vi "primary control loop.vi"(8 "loop comms in":T1, 9 "worker pool reference":T17, 10 "cmd fifo":refnum<k33>, 11 "engine out":T2={"timed loop timer source"={"Processor"=-2, "Priority"=0, "timing source dt"=0, "timer source"=refnum}, "control loop data"={"engine tag bus"={"Double"=[], "Single"=[], "I64"=[], "I32"=[], "I16"=[], "I8"=[], "U64"=[], "U32"=[], "U16"=[], "U8"=[], "Boolean"=[], "String"=[], "Array of Double"=[], "Array of Single"=[], "Array of I64"=[], "Array of I32"=[], "Array of I16"=[], "Array of I8"=[], "Array of U64"=[], "Array of U32"=[], "Array of U16"=[], "Array of U8"=[], "Array of Boolean"=[], "Array of String"=[]}, "engine schedule"={"module run flags"=[], "decimation schedule"={"decimations"=[], "offsets"=[]}}, "module information"=[]}, "status reporting"={"late? index (bool)"=-1, "late count index (U32)"=-1, "dt (ns) index (U64)"=-1, "execution time (ns) index (U64)"=-1}}) -> (0 "error out":errorcluster, 2 "desired state":T20, 3 "engine out":T2={"timed loop timer source"={"Processor"=-2, "Priority"=0, "timing source dt"=0, "timer source"=refnum}, "control loop data"={"engine tag bus"={"Double"=[], "Single"=[], "I64"=[], "I32"=[], "I16"=[], "I8"=[], "U64"=[], "U32"=[], "U16"=[], "U8"=[], "Boolean"=[], "String"=[], "Array of Double"=[], "Array of Single"=[], "Array of I64"=[], "Array of I32"=[], "Array of I16"=[], "Array of I8"=[], "Array of U64"=[], "Array of U32"=[], "Array of U16"=[], "Array of U8"=[], "Array of Boolean"=[], "Array of String"=[]}, "engine schedule"={"module run flags"=[], "decimation schedule"={"decimations"=[], "offsets"=[]}}, "module information"=[]}, "status reporting"={"late? index (bool)"=-1, "late count index (U32)"=-1, "dt (ns) index (U64)"=-1, "execution time (ns) index (U64)"=-1}})   [LabVIEW 2013, in "main engine.lvlib"]
doc: "Runs the main control timed loop of the engine."
uses:
  main engine.lvlib
  <vilib>/NI/DCAF Execution Engine Interface/Engine Runtime/Execution States.ctl
  worker library/worker comms.ctl
  worker library/worker commands.ctl
  worker library/request fifos.ctl
  worker library/recovery request.ctl
  <vilib>/NI/DCAF Module Framework/runtime/TBM module execution interface.lvclass
  <vilib>/NI/DCAF Module Framework/module configuration/TBM module configuration.lvclass
  worker library/rt fault.ctl
  <vilib>/NI/DCAF Module Framework/runtime/error classification.ctl
  worker library/response fifos.ctl
  worker library/recovery response.ctl
  <vilib>/NI/DCAF Execution Engine Interface/Engine Runtime/Fault.ctl
  Engine Data.ctl
  <vilib>/NI/Module Timing Source/timing source/TBM timing source.lvclass
  timed loop timing sources.ctl
  control loop data.ctl
  <vilib>/NI/Tag Bus/table/data table.ctl
  engine run schedule.ctl
  engine decimation schedule.ctl
  full module data.ctl
  module run state.ctl
  async executor/asynchronous executor reference.ctl
  async executor/async message to executor.ctl
  Runtime/async command notification.ctl
  Runtime/async error info.ctl
  module method data.ctl
  <vilib>/NI/Tag Bus/table/transfer specification.ctl
  <vilib>/NI/Tag Bus/tag/Data Type.ctl
  fault handling spec.ctl
  Configuration/Error Actions.ctl
  status reporting data.ctl
  loop comms.ctl
  message to engine.ctl
  message request type.ctl
  message from engine.ctl
  message response type.ctl
  <vilib>/Platform/TimedLoop/XDataNode/timing_clust.ctl
  <vilib>/Platform/TimedLoop/XDataNode/nitl_modes.ctl
  <vilib>/Platform/TimedLoop/XDataNode/wakeup.ctl
  time information.ctl
  <vilib>/NI/Tag Bus/table/transfer table data.vi
  async executor/async input data method.vi
  async executor/async process data method.vi
  async executor/async output data method.vi
  <vilib>/platform/TimedLoop/XDataNode/XDataNode.xnode
  <vilib>/Platform/TimedLoop/XDataNode/XDNodeRunTimeDep.lvlib
  <vilib>/NI/DCAF Execution Engine Interface/Engine Runtime/Engine Runtime Interface.lvclass
  <vilib>/NI/Tag Bus/table/data table.lvlib
  <vilib>/NI/Tag Bus/tag/tag descriptor.lvclass
  Configuration/Standard Engine Configuration.lvclass
  worker library/worker pool.lvlib
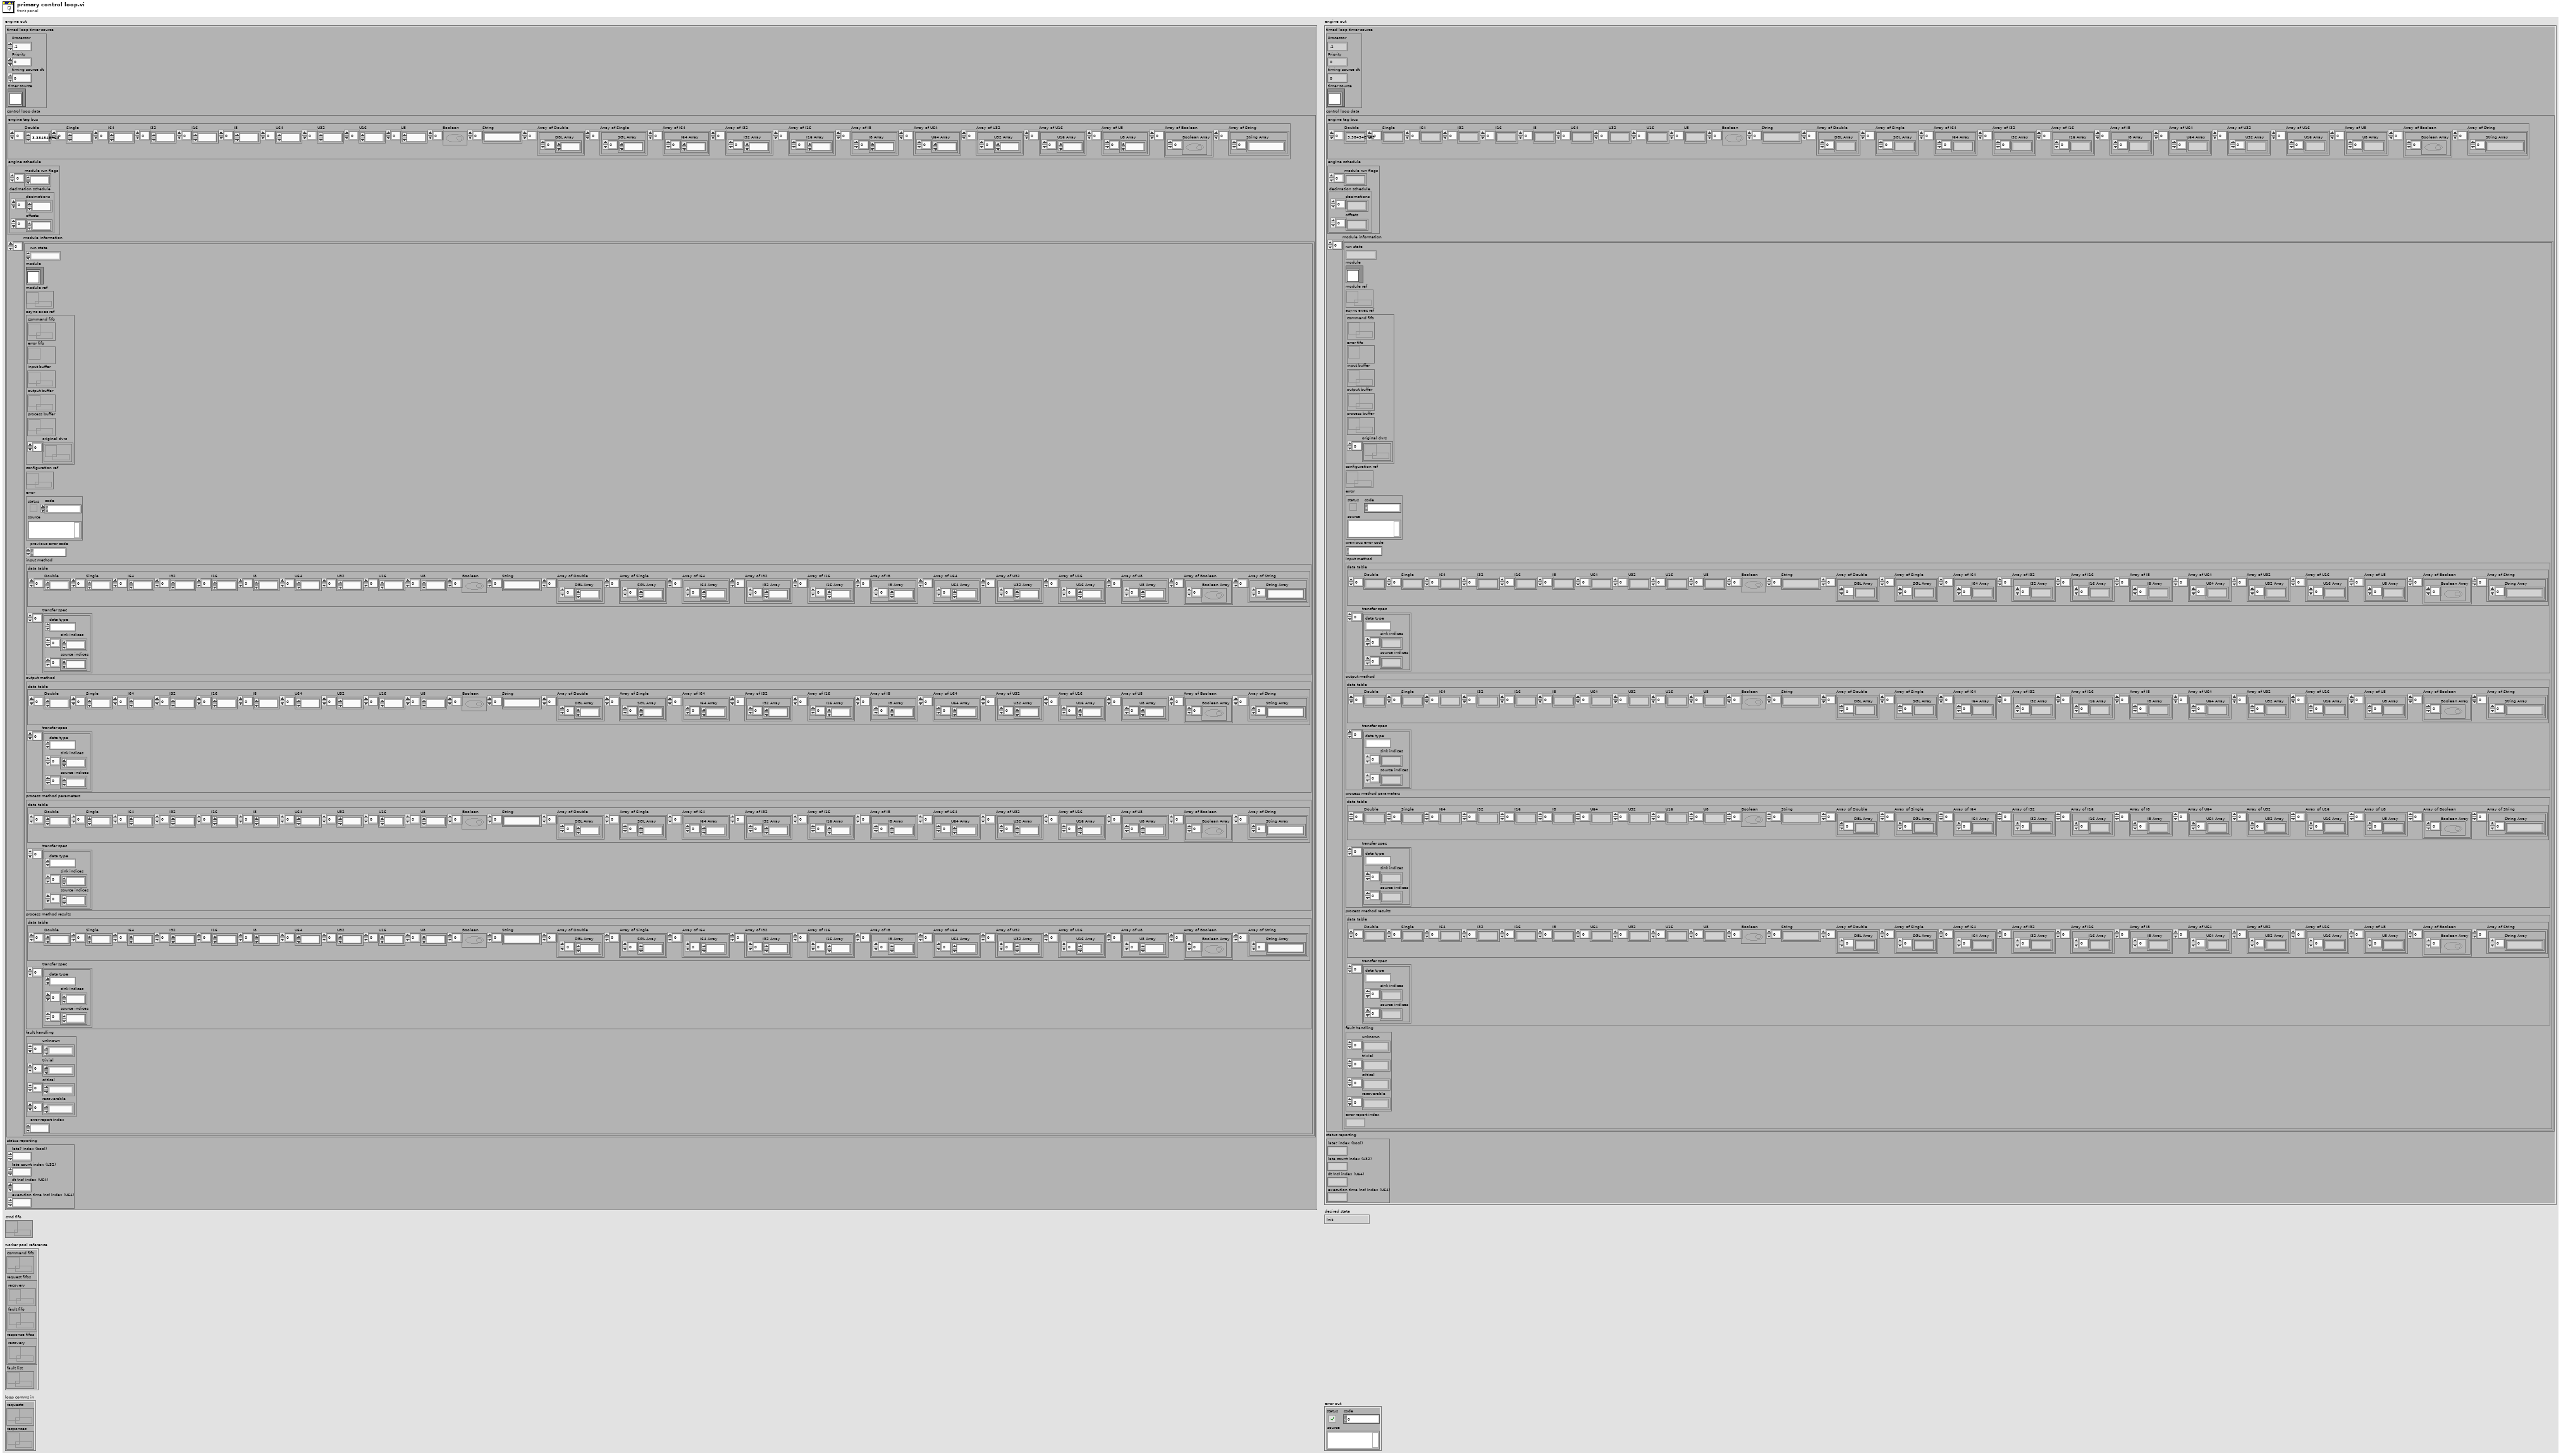
[diagram p1: front panel]
types:
  T1 = typedef "main engine.lvlib/loop comms.ctl" = cluster{"requests":refnum<k33>, "responses":refnum<k33>}
  T2 = typedef "main engine.lvlib/Engine Data.ctl" = cluster{"timed loop timer source":T3, "control loop data":T4, "status reporting":T16}
  T3 = typedef "main engine.lvlib/timed loop timing sources.ctl" = cluster{"Processor":i32, "Priority":i32, "timing source dt":u32, "timer source":refnum<class "TBM timing source.lvclass">}
  T4 = typedef "main engine.lvlib/control loop data.ctl" = cluster{"engine tag bus":T5, "engine schedule":T6, "module information":T8[]}
  T5 = typedef "tag bus.lvlib/data table.lvlib/data table.ctl" = cluster{"Double":dbl[], "Single":sgl[], "I64":i64[], "I32":i32[], "I16":i16[], "I8":i8[], "U64":u64[], "U32":u32[], "U16":u16[], "U8":u8[], "Boolean":bool[], "String":string[], "Array of Double":cluster{"DBL Array":dbl[]}[], "Array of Single":cluster{"SGL Array":sgl[]}[], "Array of I64":cluster{"I64 Array":i64[]}[], "Array of I32":cluster{"I32 Array":i32[]}[], "Array of I16":cluster{"I16 Array":i16[]}[], "Array of I8":cluster{"I8 Array":i8[]}[], "Array of U64":cluster{"U64 Array":u64[]}[], "Array of U32":cluster{"U32 Array":u32[]}[], "Array of U16":cluster{"U16 Array":u16[]}[], "Array of U8":cluster{"U8 Array":u8[]}[], "Array of Boolean":cluster{"Boolean Array":bool[]}[], "Array of String":cluster{"String Array":string[]}[]}
  T6 = typedef "main engine.lvlib/engine run schedule.ctl" = cluster{"module run flags":u8[], "decimation schedule":T7}
  T7 = typedef "main engine.lvlib/engine decimation schedule.ctl" = cluster{"decimations":u16[], "offsets":u16[]}
  T8 = typedef "main engine.lvlib/full module data.ctl" = cluster{"run state":T9, "module":refnum<class "TBM module execution interface.lvclass">, "module ref":refnum<data-value>, "async exec ref":T10, "configuration ref":refnum<data-value>, "error":errorcluster, "previous error code":i32, "input method":T11, "output method":T11, "process method parameters":T11, "process method results":T11, "fault handling":T14, "error report index ":i32}
  T9 = typedef "main engine.lvlib/module run state.ctl" = enum16{"sync", "async"}
  T10 = typedef "main engine.lvlib/asynchronous executor reference.ctl" = cluster{"command fifo":refnum<k33>, "error fifo":refnum<k33>, "input buffer":refnum<k33>, "output buffer":refnum<k33>, "process buffer":refnum<k33>, "original dvrs":refnum<data-value>[]}
  T11 = typedef "main engine.lvlib/module method data.ctl" = cluster{"data table":T5, "transfer spec":T12[]}
  T12 = typedef "tag bus.lvlib/data table.lvlib/transfer specification.ctl" = cluster{"data type":T13, "sink indices":i32[], "source indices":i32[]}
  T13 = typedef "tag bus.lvlib/tag descriptor.lvclass/Data Type.ctl" = enum16{"Double", "Single", "I64", "I32", "I16", "I8", "U64", "U32", "U16", "U8", "Boolean", "String", "Array of Double", "Array of Single", "Array of I64", "Array of I32", "Array of I16", "Array of I8", "Array of U64", "Array of U32", "Array of U16", "Array of U8", "Array of Boolean", "Array of String"}
  T14 = typedef "main engine.lvlib/fault handling spec.ctl" = cluster{"unknown":T15[], "trivial":T15[], "critical":T15[], "recoverable":T15[]}
  T15 = typedef "Standard Engine Configuration.lvclass/Error Actions.ctl" = enum16{"Clear", "Notify", "Stop Component", "Stop Engine", "Safe State", "Attempt Recovery"}
  T16 = typedef "main engine.lvlib/status reporting data.ctl" = cluster{"late? index (bool)":i32, "late count index (U32)":i32, "dt (ns) index (U64)":i32, "execution time (ns) index (U64)":i32}
  T17 = typedef "worker pool.lvlib/worker comms.ctl" = cluster{"command fifo":refnum<k33>, "request fifos":T18, "response fifos":T19, "fault list":refnum<data-value>}
  T18 = typedef "worker pool.lvlib/request fifos.ctl" = cluster{"recovery":refnum<k33>, "fault fifo":refnum<k33>}
  T19 = typedef "worker pool.lvlib/response fifos.ctl" = cluster{"recovery":refnum<k33>}
  T20 = typedef "Engine Runtime Interface.lvclass/Execution States.ctl" = enum16{"Init", "Pre-Operational", "Safe-Operational", "Operational", "Stopped"}
  T21 = typedef "main engine.lvlib/time information.ctl" = cluster{"ns since last call":u64, "finished late?":bool, "late count":u32, "iterations":u64, "ns exec time":u64}
  T22 = typedef "XDNodeRunTimeDep.lvlib/timing_clust.ctl" = cluster{"Expected End [f-1]":u64, "Actual End [f-1]":u64, "Finished Late? [f-1]":bool, "Expected End [i-1]":u64, "Actual End [i-1]":u64, "Finished Late? [i-1]":bool, "Expected Start [i]":u64, "Actual Start [i]":u64, "Expected Start [f]":u64, "Actual Start [f]":u64, "Source Name":string, "Structure Name":string, "Period":i64, "Deadline":i64, "Offset":i64, "Start":i64, "Priority":i32, "Timeout":i32, "Mode":T23, "Wakeup Reason":T24, "Error":errorcluster, "Source Type":string, "Secondary Source Type":string, "Global End Time":u64, "Global Start Time":u64, "Frame Duration":u64, "Iteration Duration":u64, "Assigned CPU":i32, "I/O Scan Engine Mode":u32}
  T23 = typedef "XDNodeRunTimeDep.lvlib/nitl_modes.ctl" = enum32{"No Change", "Process missed periods, maintain original phase", "Discard missed periods, maintain original phase", "Process missed periods, ignore original phase", "Discard missed periods, ignore original phase"}
  T24 = typedef "XDNodeRunTimeDep.lvlib/wakeup.ctl" = enum32{"Normal", "Aborted", "Asynchronous wakeup", "Timing source error", "Timed loop error", "Timeout"}
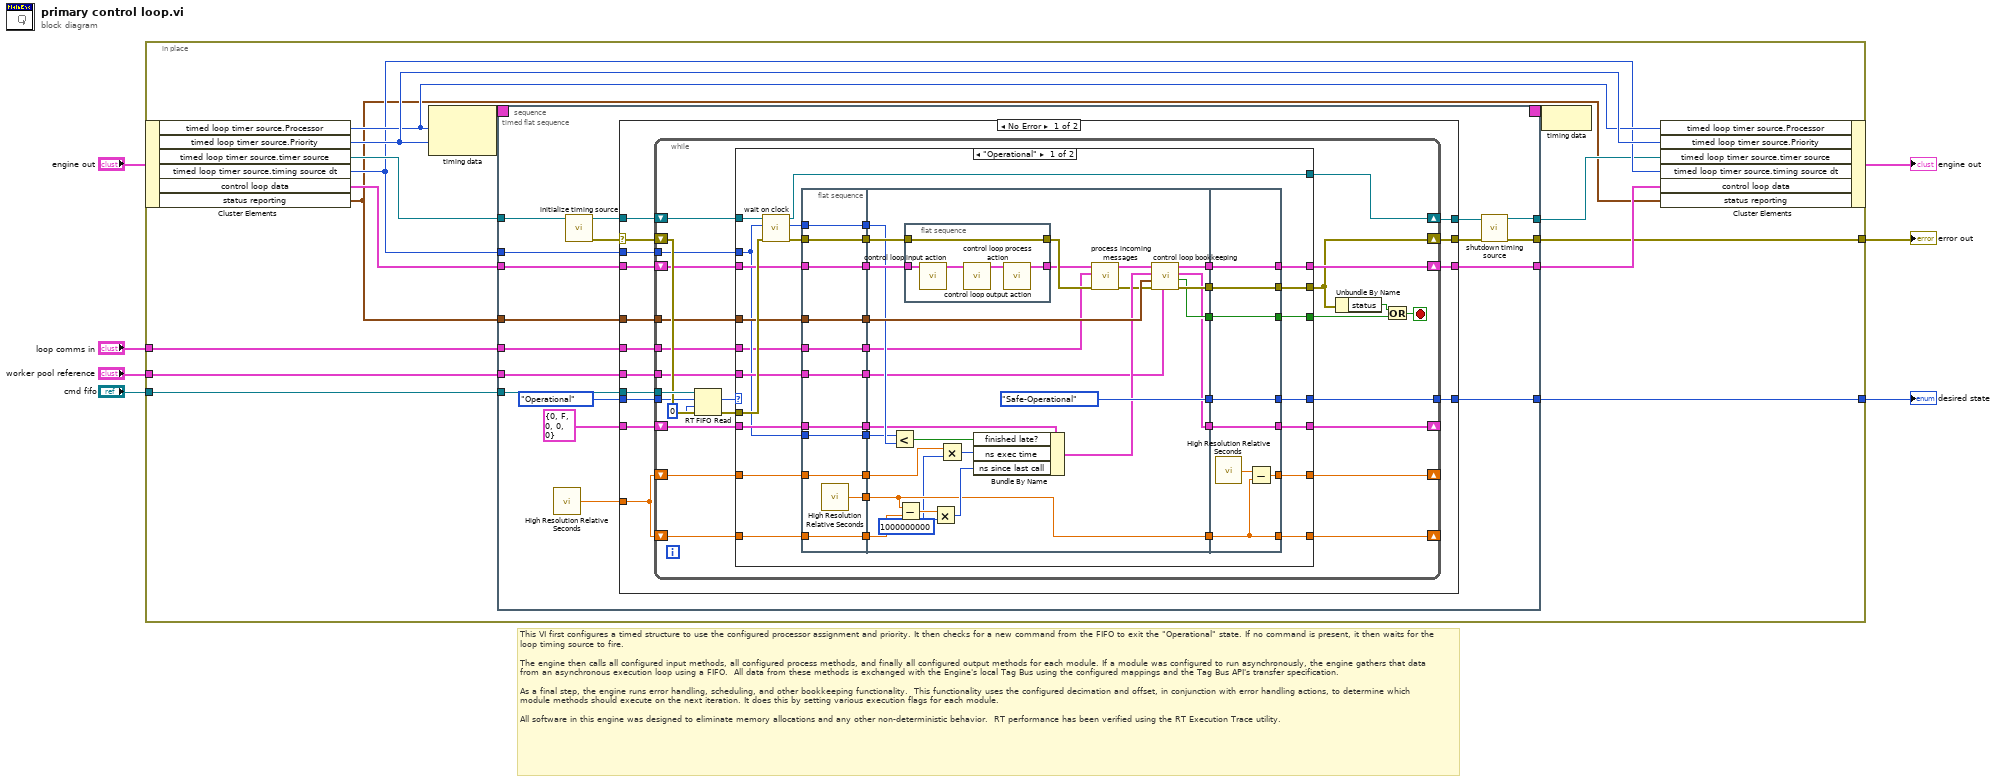
[diagram p0: block diagram]
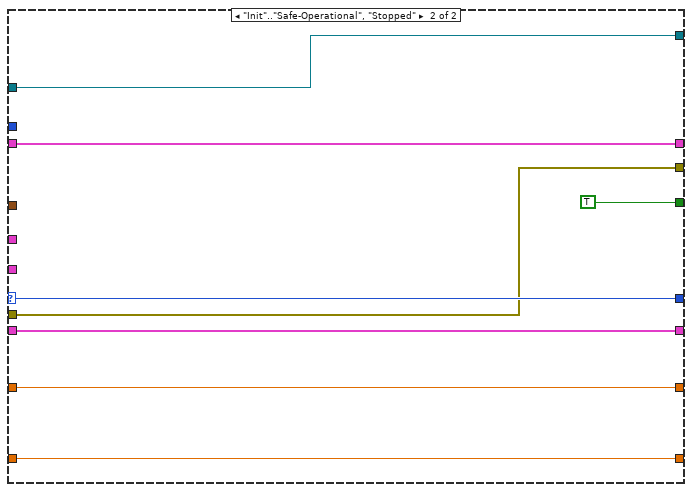
[diagram p2: hidden frame]
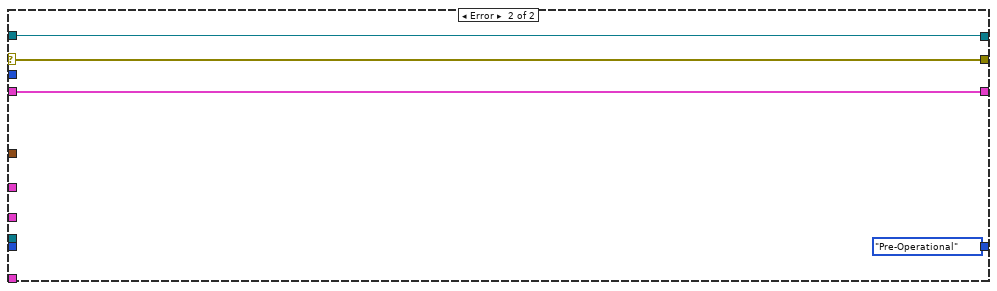
[diagram p3: hidden frame]
diagram:
  # "This VI first configures a timed structure to use the configured processor assignment and priority. It then checks for a new command from the FIFO to exit the \"Operational\" state. If no command is present, it then waits for the loop timing source to fire.   \n\nThe engine then calls all configured input methods, all configured process methods, and finally all configured output methods for each module. If a module was configured to run asynchronously, the engine gathers that data from an asynchronous execution loop using a FIFO.  All data from these methods is exchanged with the Engine's local Tag Bus using the configured mappings and the Tag Bus API's transfer specification. \n\nAs a final step, the engine runs error handling, scheduling, and other bookkeeping functionality.  This functionality uses the configured decimation and offset, in conjunction with error handling actions, to determine which module methods should execute on the next iteration. It does this by setting various execution flags for each module.\n\nAll software in this engine was designed to eliminate memory allocations and any other non-deterministic behavior.  RT performance has been verified using the RT Execution Trace utility."
  n1 = in-place {
    in-place-border: [w13] -> w5
    in-place-border: "cmd fifo" -> [w12]
    in-place-border: "worker pool reference" -> [w11]
    in-place-border: [w10] -> w2
    in-place-border: "loop comms in" -> [w8]
    n2 = in-place-cluster #1("engine out") -> ("timed loop timer source.Processor"=w17:i32, "timed loop timer source.Priority"=w18:i32, "timed loop timer source.timer source"=w20:refnum<class "TBM timing source.lvclass">, "timed loop timer source.timing source dt"=w16:u32, "control loop data"=w19:T4, "status reporting"=w9:T16)
    n3 = node-c288(w17, w18) -> (w22:T22)
    n4 = timed-sequence {
      timing: w22 -> [_]
      timing-out: [_] -> w21
      tunnel: w20 -> [w33]
      tunnel: w19 -> [w28]
      tunnel: w16 -> [w32]
      tunnel: [w31] -> w15
      tunnel: [w30] -> w13
      tunnel: [w29] -> w14
      tunnel: w12 -> [w27]
      tunnel: w11 -> [w26]
      tunnel: [w25] -> w10
      tunnel: w9 -> [w24]
      tunnel: w8 -> [w23]
      n5 = timed-flat-sequence {
        tunnel: w33 -> [w51]
        tunnel: w32 -> [w49]
        tunnel: [w42] -> w31
        tunnel: [w44] -> w30
        tunnel: [w46] -> w29
        tunnel: w28 -> [w45]
        tunnel: w27 -> [w41]
        tunnel: w26 -> [w40]
        tunnel: [w38] -> w25
        tunnel: w24 -> [w37]
        tunnel: w23 -> [w34]
        n6 = call <vilib>:"High Resolution Relative Seconds.vi"() -> ("relative seconds"=w36:dbl)
        n7 = call-dynamic "initialize timing source.vi"("timing source in"=w51) -> ("error out"=w50:errorcluster, "timing source out"=w48:refnum<class "TBM timing source.lvclass">)  [unwired: 9 in]
        n8 = case shown="No Error" w50 {
          selector: w50 -> [w64 w189]
          tunnel: w49 -> [w56 _]
          tunnel: [w65 w190] -> w43
          tunnel: w48 -> [w66 w190]
          tunnel: [w63 w189] -> w47
          tunnel: [w61 w188] -> w46
          tunnel: w45 -> [w62 w188]
          tunnel: w41 -> [w60 _]
          tunnel: w40 -> [w59 _]
          tunnel: Execution_States."Operational" ("element") -> [w58 _]
          tunnel: [w57 Execution_States."Pre-Operational"] -> w38
          tunnel: w37 -> [w55 _]
          tunnel: w36 -> [w53 _]
          tunnel: T21 {"ns since last call"=0, "finished late?"=FALSE, "late count"=0, "iterations"=0, "ns exec time"=0} ("time data") -> [w54 _]
          tunnel: w34 -> [w52 _]
          frame No Error {
            n9 = while {
              shift-right: [w82] -> w65
              shift-left: w66 -> [w83]
              shift-right: [w76] -> w63
              shift-left: w64 -> [w90]
              shift-right: [w80] -> w61
              shift-left: w62 -> [w81]
              tunnel: w60 -> [w91]
              tunnel: w59 -> [w78]
              tunnel: w58 -> [w88]
              tunnel: [w85] -> w57
              tunnel: w56 -> [w79]
              tunnel: w55 -> [w74]
              shift-right: [w72] -> _
              shift-left: w54 -> [w73]
              shift-right: [w70] -> _
              shift-left: w53 -> [w71]
              shift-right: [w69] -> _
              shift-left: w53 -> [w68]
              tunnel: w52 -> [w67]
              stop <- w77 stop-if-true
              n10 = RT FIFO Read(0:w91, 1:w88, 2:0 ("timeout in ms (0)"), 3:w90) -> (9:w87:T20, 11:w86:errorcluster)  [unwired: 3 out]
              n11 = case shown="\"Operational\"" w87 {
                selector: w87 -> [_ w186]
                tunnel: w86 -> [w127 w185]
                tunnel: [w118 w186] -> w85
                tunnel: [w120 w185] -> w76
                tunnel: [w119 TRUE] -> w84
                tunnel: w83 -> [w128 w183]
                tunnel: [w126 w183] -> w82
                tunnel: w81 -> [w125 w182]
                tunnel: [w124 w182] -> w80
                tunnel: w79 -> [w113 _]
                tunnel: w78 -> [w114 _]
                tunnel: w74 -> [w122 _]
                tunnel: w73 -> [w117 w181]
                tunnel: [w116 w181] -> w72
                tunnel: w71 -> [w115 w180]
                tunnel: [w103 w180] -> w70
                tunnel: [w96 w179] -> w69
                tunnel: w68 -> [w95 w179]
                tunnel: w67 -> [w92 _]
                frame "Operational" {
                  n12 = call-dynamic "wait on clock.vi"("error in"=w127, "dt"=w113, "timing source in"=w128) -> ("error out"=w123:errorcluster, "ticks since last call"=w121:u32, "timing source out"=w126:refnum<class "TBM timing source.lvclass">)  [unwired: 6 in]
                  n13 = flat-sequence {
                    tunnel: w114 -> [w132]
                    tunnel: w115 -> [w133]
                    tunnel: w117 -> [w134]
                    tunnel: w113 -> [w135]
                    tunnel: w121 -> [w136]
                    tunnel: w122 -> [w137]
                    tunnel: w123 -> [w138]
                    tunnel: w125 -> [w139]
                    tunnel: [w139] -> w112
                    tunnel: [w138] -> w111
                    tunnel: [w137] -> w110
                    tunnel: [w136] -> w109
                    tunnel: [w135] -> w108
                    tunnel: [w134] -> w107
                    tunnel: [w133] -> w106
                    tunnel: [w131] -> w105
                    tunnel: [w132] -> w104
                    tunnel: w95 -> [w130]
                    tunnel: [w130] -> w94
                    tunnel: [w129] -> w93
                    tunnel: w92 -> [w129]
                    tunnel: w112 -> [w165]
                    tunnel: w111 -> [w163]
                    tunnel: w110 -> [w162]
                    tunnel: w109 -> [w161]
                    tunnel: w108 -> [w160]
                    tunnel: w107 -> [w156]
                    tunnel: w106 -> [w152]
                    tunnel: w105 -> [w148]
                    tunnel: w104 -> [w149]
                    tunnel: [w164] -> w102
                    tunnel: [w159] -> w101
                    tunnel: [w158] -> w100
                    tunnel: [Execution_States."Safe-Operational"] -> w99
                    tunnel: [w155] -> w98
                    tunnel: [w148] -> w97
                    tunnel: w94 -> [w145]
                    tunnel: w93 -> [w140]
                    tunnel: [w172] -> w103
                    tunnel: [w174] -> w116
                    tunnel: [w175] -> w118
                    tunnel: [w176] -> w119
                    tunnel: [w177] -> w120
                    tunnel: [w178] -> w124
                    tunnel: w102 -> [w178]
                    tunnel: w101 -> [w177]
                    tunnel: w100 -> [w176]
                    tunnel: w99 -> [w175]
                    tunnel: w98 -> [w174]
                    tunnel: w97 -> [w172]
                    tunnel: [w171] -> w96
                    frame #0 {
                      n14 = call <vilib>:"High Resolution Relative Seconds.vi"() -> ("relative seconds"=w131:dbl)
                    }
                    frame #1 {
                      w146 = 1000000000
                      n15 = Less?(x=w160, y=w161) -> (x < y?=w153:bool)
                      n16 = Subtract(x=w148, y=w152) -> (x-y=w151:dbl)
                      n17 = flat-sequence {
                        tunnel: w165 -> [w168]
                        tunnel: [w167] -> w143
                        tunnel: w163 -> [w166]
                        tunnel: [w166] -> w144
                        frame #0 {
                          n18 = call "control loop input action.vi"("control loop data in"=w168) -> ("control loop data out"=w170:T4)  [unwired: 10 in]
                          n19 = call "control loop process action.vi"("control loop data in"=w170) -> ("control loop data out"=w169:T4)  [unwired: 10 in]
                          n20 = call "control loop output action.vi"("control loop data in"=w169) -> ("control loop data out"=w167:T4)  [unwired: 10 in]
                        }
                      }
                      n21 = Multiply(x=w151, y=w146) -> (x*y=w150:u64)
                      n22 = Multiply(x=w145, y=w146) -> (x*y=w147:u64)
                      n23 = Bundle By Name(cluster=w156, "finished late?"=w153, "ns exec time"=w147, "ns since last call"=w150) -> (w154:T21)
                      n24 = call "process incoming messages.vi"("error in"=w144, "loop comms in"=w140, "control loop data in"=w143) -> ("error out"=w142:errorcluster, "control loop data out"=w141:T4)  [unwired: 7 in]
                      n25 = call "control loop bookkeeping.vi"("worker pool reference"=w149, "engine error in"=w142, "status reporting in"=w162, "time data in"=w154, "control loop data in"=w141) -> ("engine error out"=w159:errorcluster, "safe state?"=w158:bool, "time data out"=w155:T21, "control loop data out"=w164:T4)  [unwired: 3 in]
                    }
                    frame #2 {
                      n26 = call <vilib>:"High Resolution Relative Seconds.vi"() -> ("relative seconds"=w173:dbl)
                      n27 = Subtract(x=w173, y=w172) -> (x-y=w171:dbl)
                    }
                  }
                }
                frame "Init".."Safe-Operational", "Stopped" {
                }
              }
              n28 = Unbundle By Name(w76) -> ("status"=w75:bool)
              n29 = Or(x=w75, y=w84) -> (x .or. y?=w77:bool)
            }
          }
          frame Error {
          }
        }
        n30 = call-dynamic "shutdown timing source.vi"("error in"=w47, "timing source in"=w43) -> ("error out"=w44:errorcluster, "timing source out"=w42:refnum<class "TBM timing source.lvclass">)  [unwired: 8 in]
      }
    }
    n31 = node-c288(w21) -> ()
    n32 = in-place-cluster #1("timed loop timer source.Processor"=w17, "timed loop timer source.Priority"=w18, "timed loop timer source.timer source"=w15, "timed loop timer source.timing source dt"=w16, "control loop data"=w14, "status reporting"=w9) -> (→"engine out":T2)
  }
  "desired state" <- w2
  "error out" <- w5
